vi "All Motor Controllers.vi"() -> ()   [LabVIEW 2017]
uses:
  <vilib>/Rock Robotics/SystemInterfaces/DIO/FPGA_DIOPWMChannel.ctl
  <vilib>/Rock Robotics/SystemInterfaces/DIO/FPGA_DIORelayChannel.ctl
  <vilib>/Rock Robotics/WPI/Solenoid/WPI_SolenoidChannel.ctl
  <vilib>/Rock Robotics/WPI/Relay/WPI_RelayValue.ctl
  <vilib>/Rock Robotics/WPI/Relay/WPI_RelayDirection.ctl
  <vilib>/Rock Robotics/WPI/Solenoid/WPI_SolenoidValue.ctl
  <vilib>/Rock Robotics/WPI/MotorControl/WPI_MotorControlOpen VictorSP.vi
  <vilib>/Rock Robotics/WPI/MotorControl/WPI_MotorControlOpen SPARK.vi
  <vilib>/Rock Robotics/WPI/MotorControl/WPI_MotorControlOpen TalonSRX.vi
  <vilib>/Rock Robotics/WPI/Solenoid/WPI_SolenoidOpenDouble.vi
  <vilib>/Rock Robotics/WPI/Solenoid/WPI_SolenoidSetEnum.vi
panel:
  in  "Reverse":bool
  in  "Forward":bool
  in  "RelayValue":T1
  in  "Compressor":bool
  in  "Reverse Solenoid Channel":T2=enum."Solenoid 1"
  in  "Forward Solenoid Channel":T2
  in  "Relay Channel":T3
  in  "s 8":bool=TRUE
  in  "s 7":bool=TRUE
  in  "s 6":bool=TRUE
  in  "s 5":bool=TRUE
  in  "s 4":bool=TRUE
  in  "s 3":bool=TRUE
  in  "s 2":bool=TRUE
  in  "s":bool=TRUE
  in  "Speed (-1 to 1)":dbl(slide) min=-1.0 max=1.0 step=0.1 scale=-1.0..1.0 scale format="%#.3f"
  in  "Speed Test Type":T4(ring)=enum."Variable"
  in  "Victor SPX":T5=enum."PWM 7"
  in  "Talon SRX 4":T5=enum."PWM 4"
  in  "Talon SRX 5":T5=enum."PWM 5"
  in  "SPARK":T5=enum."PWM 6"
  in  "Right Rear Mecanum":T5=enum."PWM 3"
  in  "Right Front Mecanum":T5=enum."PWM 2"
  in  "Left Rear Mecanum":T5=enum."PWM 1"
  in  "stop":bool
  in  "Left Front Mecanum":T5
  # "Configure inputs before running."
  # "This can be set while running."
  # "Configure inputs before running."
  # "Select Device Action"
  # "Motor Enable."
  # "This program requires the Driver Station to be running with Teleoperated Enabled."
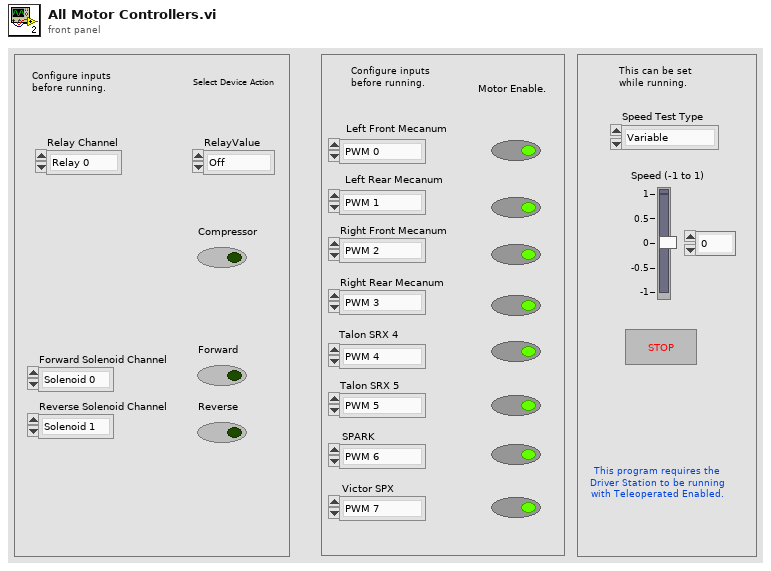
[diagram p1: front panel]
types:
  T1 = typedef "WPI_RelayValue.ctl" = enum16{"Off", "On", "Forward", "Reverse"}
  T2 = typedef "WPI_SolenoidChannel.ctl" = enum8{"Solenoid 0", "Solenoid 1", "Solenoid 2", "Solenoid 3", "Solenoid 4", "Solenoid 5", "Solenoid 6", "Solenoid 7", "Invalid"}
  T3 = typedef "FPGA_DIORelayChannel.ctl" = enum8{"Relay 0", "Relay 1", "Relay 2", "Relay 3", "Invalid"}
  T4 = enum16{"Idle", "Variable", "Forward Slow", "Reverse Slow", "Forward Full", "Reverse Full"}
  T5 = typedef "FPGA_DIOPWMChannel.ctl" = enum8{"PWM 0", "PWM 1", "PWM 2", "PWM 3", "PWM 4", "PWM 5", "PWM 6", "PWM 7", "PWM 8", "PWM 9", "PWM MXP 0", "PWM MXP 1", "PWM MXP 2", "PWM MXP 3", "PWM MXP 4", "PWM MXP 5", "PWM MXP 6", "PWM MXP 7", "PWM MXP 8", "PWM MXP 9", "Invalid"}
  T6 = typedef "WPI_RelayDirection.ctl" = enum16{"Both directions", "Forward only", "Reverse only"}
  T7 = typedef "WPI_MotorControlDeviceRef.ctl" = cluster{"DeviceStatus":errorcluster, "Type":T8, "PWM":cluster{"PWM Channel":T5, "DeadBand":T9}, "CAN":cluster{"Device Number":u8, "SetOutput VI Ref":variant, "GetOutput VI Ref":variant, "Enable VI Ref":variant, "Disable VI Ref":variant, "Data":variant}, "Invert":bool, "DIO PWM":cluster{"PWM \"Enable\" Channel":T5, "DIOChannel":T10, "PWM Rate":dbl}}
  T8 = typedef "WPI_MotorControlType.ctl" = enum16{"PWM", "CAN", "DIO PWM"}
  T9 = typedef "WPI_PWMDeadband.ctl" = cluster{"Name":string, "maxPositivePwm":i32, "minPositivePwm":i32, "centerPwm":i32, "maxNegativePwm":i32, "minNegativePwm":i32, "angularRange":u16}
  T10 = typedef "FPGA_DIOChannel.ctl" = enum8{"DIO 0", "DIO 1", "DIO 2", "DIO 3", "DIO 4", "DIO 5", "DIO 6", "DIO 7", "DIO 8", "DIO 9", "DIO MXP 0", "DIO MXP 1", "DIO MXP 2", "DIO MXP 3", "DIO MXP 4", "DIO MXP 5", "DIO MXP 6", "DIO MXP 7", "DIO MXP 8", "DIO MXP 9", "DIO MXP 10", "DIO MXP 11", "DIO MXP 12", "DIO MXP 13", "DIO MXP 14", "DIO MXP 15", "SPI Port CS1", "SPI Port CS2", "SPI Port CS3", "SPI Port MISO", "SPI Port MOSI", "Invalid"}
  T11 = typedef "WPI_CompressorDevRef.ctl" = cluster{"DevStatus":errorcluster, "Pneumatics Control Module":u8}
  T12 = typedef "WPI_RelayDevRef.ctl" = cluster{"DevStatus":errorcluster, "Relay Channel":T3, "Relay Direction":T6}
  T13 = typedef "WPI_SolenoidDevRef.ctl" = cluster{"DevStatus":errorcluster, "Pneumatics Control Module":u8, "Forward Solenoid Channel":T2, "Reverse Solenoid Channel":T2}
  T14 = typedef "WPI_SolenoidValue.ctl" = enum16{"Off", "On", "Forward", "Reverse"}
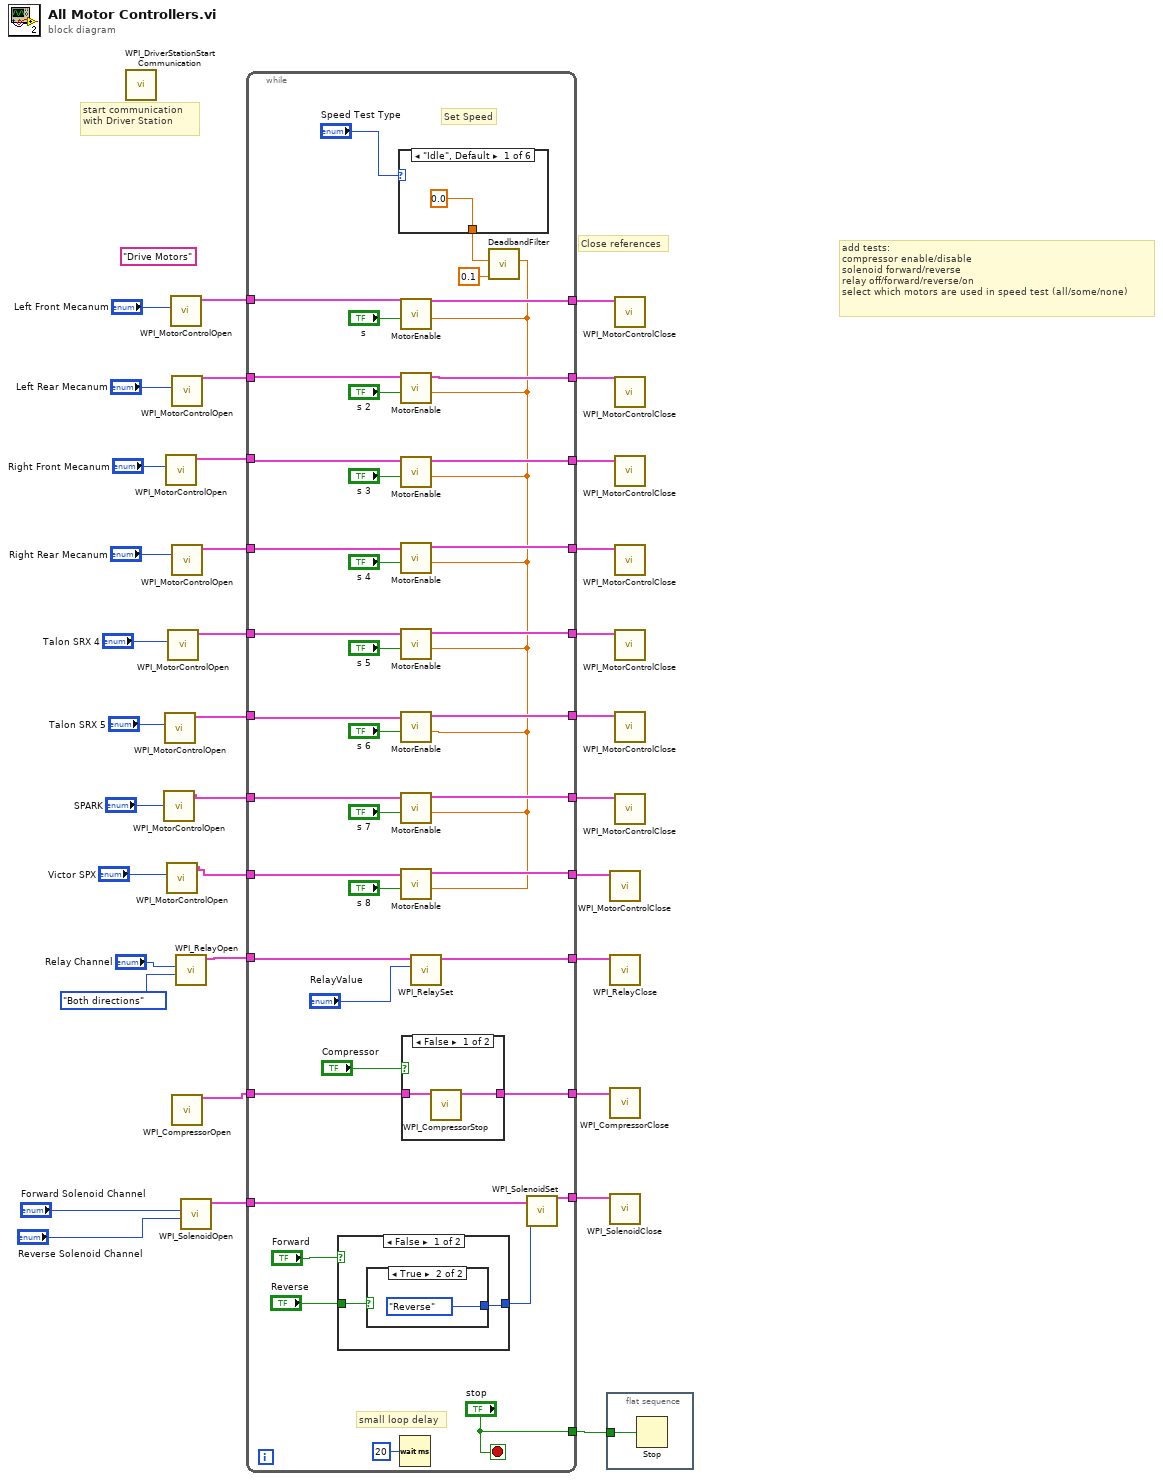
[diagram p0: block diagram]
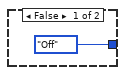
[diagram p2: hidden frame]
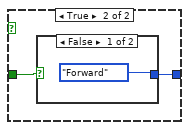
[diagram p3: hidden frame]
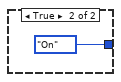
[diagram p4: hidden frame]
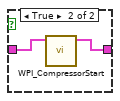
[diagram p5: hidden frame]
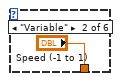
[diagram p6: hidden frame]
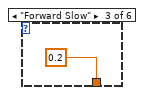
[diagram p7: hidden frame]
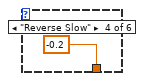
[diagram p8: hidden frame]
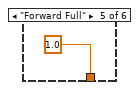
[diagram p9: hidden frame]
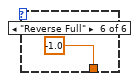
[diagram p10: hidden frame]
diagram:
  (unwired) "Drive Motors" ("refnum name")
  # "add tests:\ncompressor enable/disable\nsolenoid forward/reverse\nrelay off/forward/reverse/on\nselect which motors are used in speed test (all/some/none)"
  # "start communication with Driver Station"
  # "Close references"
  n1 = call <vilib>:"WPI_DriverStationStart Communication.vi"() -> ()  [unwired: 2 in, 10 out]
  n2 = call-poly <vilib>:"WPI_MotorControlOpen.vi"("PWM Channel"="SPARK") -> ("MotorControlDeviceRef"=w16:T7)  [unwired: 9 in, 1 out]
  n3 = call-poly <vilib>:"WPI_MotorControlOpen.vi"("PWM Channel"="Talon SRX 5") -> ("MotorControlDeviceRef"=w15:T7)  [unwired: 9 in, 1 out]
  n4 = call-poly <vilib>:"WPI_MotorControlOpen.vi"("PWM Channel"="Right Front Mecanum") -> ("MotorControlDeviceRef"=w28:T7)  [unwired: 9 in, 1 out]
  n5 = call-poly <vilib>:"WPI_MotorControlOpen.vi"("PWM Channel"="Victor SPX") -> ("MotorControlDeviceRef"=w12:T7)  [unwired: 9 in, 1 out]
  n6 = call-poly <vilib>:"WPI_MotorControlOpen.vi"("PWM Channel"="Talon SRX 4") -> ("MotorControlDeviceRef"=w14:T7)  [unwired: 9 in, 1 out]
  n7 = call-poly <vilib>:"WPI_MotorControlOpen.vi"("PWM Channel"="Left Front Mecanum") -> ("MotorControlDeviceRef"=w34:T7)  [unwired: 3 in, 7 out]
  n8 = call-poly <vilib>:"WPI_MotorControlOpen.vi"("PWM Channel"="Left Rear Mecanum") -> ("MotorControlDeviceRef"=w30:T7)  [unwired: 3 in, 7 out]
  n9 = call-poly <vilib>:"WPI_MotorControlOpen.vi"("PWM Channel"="Right Rear Mecanum") -> ("MotorControlDeviceRef"=w20:T7)  [unwired: 9 in, 1 out]
  n10 = call <vilib>:"WPI_CompressorOpen.vi"() -> ("CompressorDevRef"=w6:T11)  [unwired: 14 in, 1 out]
  n11 = call <vilib>:"WPI_RelayOpen.vi"("Relay Direction"=WPI_RelayDirection."Both directions", "Relay Channel"="Relay Channel") -> ("RelayDevRef"=w2:T12)  [unwired: 8 in, 1 out]
  n12 = call-poly <vilib>:"WPI_SolenoidOpen.vi"("Reverse Solenoid Channel"="Reverse Solenoid Channel", "Forward Solenoid Channel"="Forward Solenoid Channel") -> ("SolenoidDevRef"=w4:T13)  [unwired: 8 in, 1 out]
  n13 = while {
    tunnel: w34 -> [w72]
    tunnel: [w71] -> w33
    tunnel: ["stop"] -> w32
    tunnel: w30 -> [w66]
    tunnel: [w55] -> w29
    tunnel: w28 -> [w65]
    tunnel: [w54] -> w27
    tunnel: w20 -> [w64]
    tunnel: w14 -> [w63]
    tunnel: w15 -> [w60]
    tunnel: w16 -> [w59]
    tunnel: [w53] -> w26
    tunnel: [w52] -> w25
    tunnel: [w51] -> w24
    tunnel: [w50] -> w23
    tunnel: w12 -> [w57]
    tunnel: [w56] -> w11
    tunnel: w6 -> [w48]
    tunnel: [w47] -> w5
    tunnel: w4 -> [w43]
    tunnel: [w42] -> w3
    tunnel: w2 -> [w40]
    tunnel: [w39] -> w1
    stop <- "stop" stop-if-true
    # "small loop delay"
    # "Set Speed"
    n14 = case shown="False" "Forward" {
      tunnel: "Reverse" -> [w78 w82]
      tunnel: [w77 w81] -> w46
      frame False {
        n15 = case shown="True" w78 {
          tunnel: [WPI_SolenoidValue."Off" ("Value") WPI_SolenoidValue."Reverse" ("Value")] -> w77
          frame False {
          }
          frame True {
          }
        }
      }
      frame True {
        n16 = case shown="False" w82 {
          tunnel: [WPI_SolenoidValue."Forward" ("Value") WPI_SolenoidValue."On" ("Value")] -> w81
          frame False {
          }
          frame True {
          }
        }
      }
    }
    n17 = case shown="\"Idle\", Default" "Speed Test Type" {
      tunnel: [0.0 ("Speed (-1 to 1)") "Speed (-1 to 1)" 0.2 ("Speed (-1 to 1)") -0.2 ("Speed (-1 to 1)") 1.0 ("Speed (-1 to 1)") -1.0 ("Speed (-1 to 1)")] -> w37
      frame "Idle", Default {
      }
      frame "Variable" {
      }
      frame "Forward Slow" {
      }
      frame "Reverse Slow" {
      }
      frame "Forward Full" {
      }
      frame "Reverse Full" {
      }
    }
    n18 = Wait (ms)(milliseconds to wait=u32 20) -> ()  [unwired: 1 out]
    n19 = case shown="False" "Compressor" {
      tunnel: w48 -> [w86 w88]
      tunnel: [w85 w87] -> w47
      frame False {
        n20 = call <vilib>:"WPI_CompressorStop.vi"("CompressorDevRef"=w86) -> ("CompressorDevRef"=w85:T11)  [unwired: 9 in, 1 out]
      }
      frame True {
        n21 = call <vilib>:"WPI_CompressorStart.vi"("CompressorDevRef"=w88) -> ("CompressorDevRef"=w87:T11)  [unwired: 9 in, 1 out]
      }
    }
    n22 = call <vilib>:"WPI_RelaySet.vi"("RelayValue"="RelayValue", "RelayDevRef"=w40) -> ("RelayDevRef"=w39:T12)  [unwired: 8 in, 1 out]
    n23 = call "DeadbandFilter.vi"("guardband value"=0.1, "JoystickAxis"=w37) -> ("FilteredJoystickAxis"=w38:dbl)  [unwired: 9 in]
    n24 = call "MotorEnable.vi"("t"=w38, "s"="s", "MotorControlDevRef"=w72) -> ("MotorControlDevRef 2"=w71:T7)  [unwired: 8 in]
    n25 = call "MotorEnable.vi"("t"=w38, "s"="s 2", "MotorControlDevRef"=w66) -> ("MotorControlDevRef 2"=w55:T7)  [unwired: 8 in]
    n26 = call "MotorEnable.vi"("t"=w38, "s"="s 3", "MotorControlDevRef"=w65) -> ("MotorControlDevRef 2"=w54:T7)  [unwired: 8 in]
    n27 = call "MotorEnable.vi"("t"=w38, "s"="s 4", "MotorControlDevRef"=w64) -> ("MotorControlDevRef 2"=w53:T7)  [unwired: 8 in]
    n28 = call "MotorEnable.vi"("t"=w38, "s"="s 5", "MotorControlDevRef"=w63) -> ("MotorControlDevRef 2"=w52:T7)  [unwired: 8 in]
    n29 = call "MotorEnable.vi"("t"=w38, "s"="s 6", "MotorControlDevRef"=w60) -> ("MotorControlDevRef 2"=w51:T7)  [unwired: 8 in]
    n30 = call "MotorEnable.vi"("t"=w38, "s"="s 7", "MotorControlDevRef"=w59) -> ("MotorControlDevRef 2"=w50:T7)  [unwired: 8 in]
    n31 = call "MotorEnable.vi"("t"=w38, "s"="s 8", "MotorControlDevRef"=w57) -> ("MotorControlDevRef 2"=w56:T7)  [unwired: 8 in]
    n32 = call-poly <vilib>:"WPI_SolenoidSet.vi"("Value"=w46, "SolenoidDevRef"=w43) -> ("SolenoidDevRef"=w42:T13)  [unwired: 8 in, 1 out]
  }
  n33 = flat-sequence {
    tunnel: w32 -> [w95]
    frame #0 {
      n34 = Stop(stop? (T)=w95) -> ()
    }
  }
  n35 = call <vilib>:"WPI_MotorControlClose.vi"("MotorControlDevRef"=w11) -> ()  [unwired: 1 in, 10 out]
  n36 = call <vilib>:"WPI_RelayClose.vi"("RelayDevRef"=w1) -> ()  [unwired: 10 in, 1 out]
  n37 = call <vilib>:"WPI_CompressorClose.vi"("CompressorDevRef"=w5) -> ()  [unwired: 10 in, 1 out]
  n38 = call <vilib>:"WPI_SolenoidClose.vi"("SolenoidDevRef"=w3) -> ()  [unwired: 10 in, 1 out]
  n39 = call <vilib>:"WPI_MotorControlClose.vi"("MotorControlDevRef"=w33) -> ()  [unwired: 1 in, 10 out]
  n40 = call <vilib>:"WPI_MotorControlClose.vi"("MotorControlDevRef"=w29) -> ()  [unwired: 1 in, 10 out]
  n41 = call <vilib>:"WPI_MotorControlClose.vi"("MotorControlDevRef"=w27) -> ()  [unwired: 1 in, 10 out]
  n42 = call <vilib>:"WPI_MotorControlClose.vi"("MotorControlDevRef"=w26) -> ()  [unwired: 1 in, 10 out]
  n43 = call <vilib>:"WPI_MotorControlClose.vi"("MotorControlDevRef"=w25) -> ()  [unwired: 1 in, 10 out]
  n44 = call <vilib>:"WPI_MotorControlClose.vi"("MotorControlDevRef"=w24) -> ()  [unwired: 1 in, 10 out]
  n45 = call <vilib>:"WPI_MotorControlClose.vi"("MotorControlDevRef"=w23) -> ()  [unwired: 1 in, 10 out]
